vi "Create Annulus from Rectangle.vi"(11 "Rectangle ltrb":dbl[](array[numeric])) -> (3 "ROI Descriptor":T1 {"Contours"."Type" items=["No Selection", "Point", "Line", "Rectangle", "Oval", "Polygon", "Freehand Region", "Annulus", "Unused2", "Unused3", "Broken Line", "Freehand Line", "Rotated Rectangle"]})   [LabVIEW 2013]
doc: "Build an annulus RIO centered within the rectangle. Use half the width for the outer radius and zero for the inner one. Set angles to be a full circle."
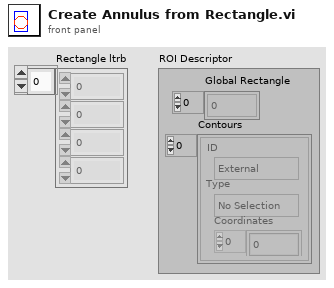
[diagram p1: front panel]
types:
  T1 = typedef "ROI Descriptor" = cluster{"Global Rectangle":i32[], "Contours":cluster{"ID":enum32{"External", "Internal"}, "Type":u32, "Coordinates":i32[]}[]}
  T2 = typedef "IMAQ Circle" = cluster{"Center X":i32, "Center Y":i32, "Inner Radius":i32, "Outer Radius":i32, "Start Angle":dbl, "End Angle":dbl}
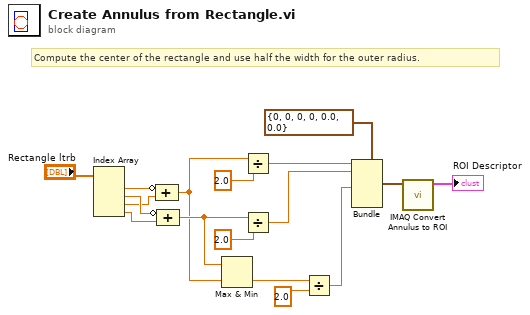
[diagram p0: block diagram]
diagram:
  # "Compute the center of the rectangle and use half the width for the outer radius."
  n1 = Index Array(array="Rectangle ltrb") -> (element #1=w3:dbl, element #2=w5:dbl, element #3=w2:dbl, element #4=w6:dbl)  [unwired: 4 in]
  n2 = Compound Arithmetic op=ADD(invert w3, w2) -> (w1:dbl)
  n3 = Compound Arithmetic op=ADD(invert w5, w6) -> (w4:dbl)
  n4 = Max & Min(x=w4, y=w1) -> (min(x,y)=w9:dbl)  [unwired: 1 out]
  n5 = Divide(x=w1, y=2.0) -> (x/y=w11:dbl)
  n6 = Divide(x=w4, y=2.0) -> (x/y=w10:dbl)
  n7 = Divide(x=w9, y=2.0) -> (x/y=w8:dbl)
  n8 = Bundle(cluster=T2 {"Center X"=0, "Center Y"=0, "Inner Radius"=0, "Outer Radius"=0, "Start Angle"=0.0, "End Angle"=0.0} ("Annulus"), "Center X"=w11, "Center Y"=w10, "Outer Radius"=w8) -> (w16:T2)  [unwired: 3 in]
  n9 = call "IMAQ Convert Annulus to ROI"("Annulus"=w16) -> ("ROI Descriptor"=→"ROI Descriptor":T1)  [unwired: 8 in, 1 out]
